vi "ReadConsiderCorrections.vi"(8 "error in":errorcluster, 11 "HP4284A.lvclass in":refnum<class "HP4284A.lvclass">) -> (0 "error out":errorcluster, 1 "Consider SC":bool, 2 "Consider OC":bool, 3 "HP4284A.lvclass  out":refnum<class "HP4284A.lvclass">)   [LabVIEW 2018, in "HP4284A.lvclass"]
uses:
  HP4284A.lvclass
  HP4284A.lvclass/HP4284A.ctl
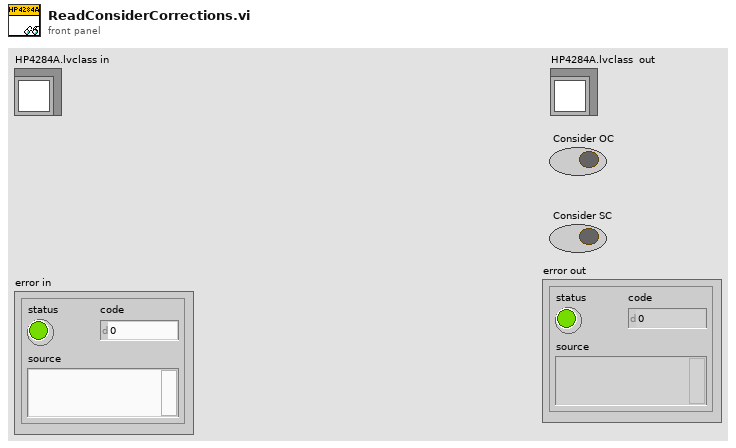
[diagram p1: front panel]
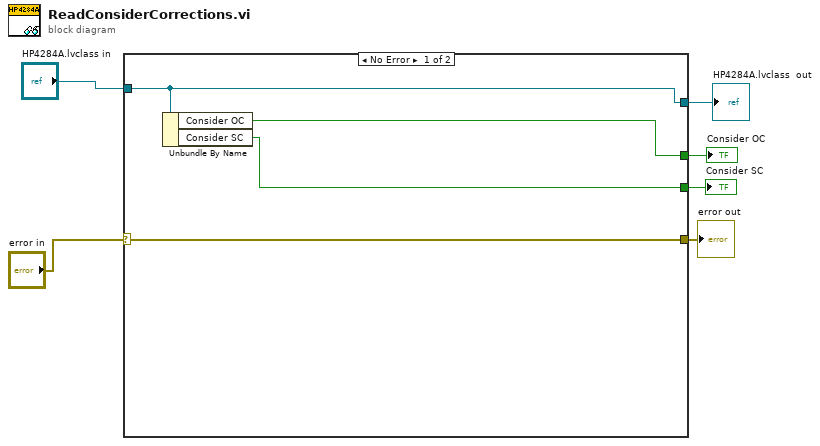
[diagram p0: block diagram]
diagram:
  n1 = case shown="No Error" "error in" {
    selector: "error in" -> [w10 w12]
    tunnel: "HP4284A.lvclass in" -> [w9 w11]
    tunnel: [w9 w11] -> w5
    tunnel: [w10 w12] -> w3
    tunnel: [w8 _] -> w2
    tunnel: [w7 _] -> w1
    frame No Error {
      n2 = Unbundle By Name(w9) -> ("Consider OC"=w8:bool, "Consider SC"=w7:bool)
    }
    frame Error {
    }
  }
  "Consider OC" <- w2
  "HP4284A.lvclass  out" <- w5
  "error out" <- w3
  "Consider SC" <- w1
